vi "XIPIN_Color_Filter_Array_Interpolation_7_0.vi"   [LabVIEW 2017]
doc: "The Xilinx LogiCORE Color Filter Array Interpolation Core reconstructs RGB data from color image sensors equipped with a Bayer Color Filter Array.\n------------------------------------\n<b>Need License</b> : Yes\n<b>Interface</b> : AXI4 AXI4-Stream"
uses:
  <vilib>/rvi/XilinxIP/XIPIN_XNode/niFpgaXIPIN.xnode
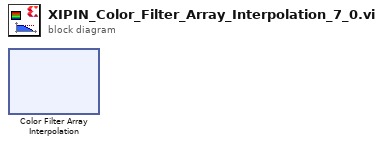
[diagram p0: block diagram]
diagram:
  n1 = xnode ("Color Filter Array Interpolation")() -> ()
